vi "耐久性测试.vi"(6 "Bool引用句柄":refnum<vi>, 9 "输出簇 2":T4, 10 "输出簇":T4, 11 "事件注册引用句柄 2":refnum<event-registration>) -> ()   [LabVIEW 2020]
uses:
  <vilib>/Utility/miscctls.llb/LVRectTypeDef.ctl
  Windows/System32/user32.dll
panel:
  in  "布尔 3":T1
  in  "布尔 2":T2
  in  "布尔":T3
  out "数值 2":dbl format="%#_2f V"
  out "数值":dbl format="%#_2f A"
  out "电流":dbl[](graph)
  out "电压":dbl[](graph)
  # "耐久性测试"
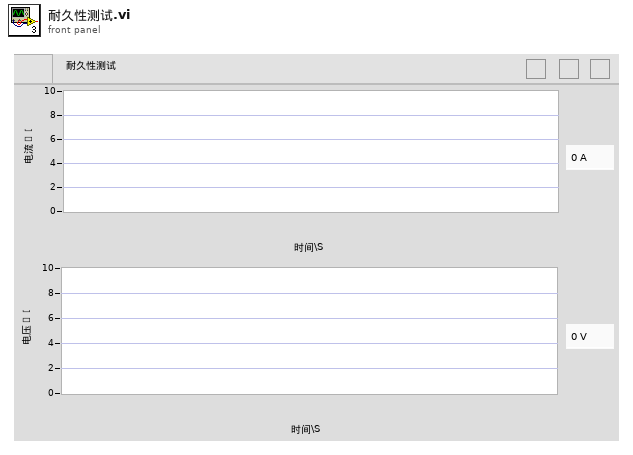
[diagram p1: front panel]
types:
  T1 = typedef "控件关闭.ctl" = bool
  T2 = typedef "控件最小化.ctl" = bool
  T3 = typedef "控件最大化.ctl" = bool
  T4 = cluster{"电流1":refnum<vi>, "电流2":refnum<vi>, "电流3":refnum<vi>, "电流4":refnum<vi>}
  T5 = typedef "LVRectTypeDef.ctl" = cluster{"Left":i16, "Top":i16, "Right":i16, "Bottom":i16}
  T6 = typedef "LVPoint32TypeDef.ctl" = cluster{"Horizontal":i32, "Vertical":i32}
  T7 = enum32{"Invalid", "Standard", "Closed", "Hidden", "Minimized", "Maximized"}
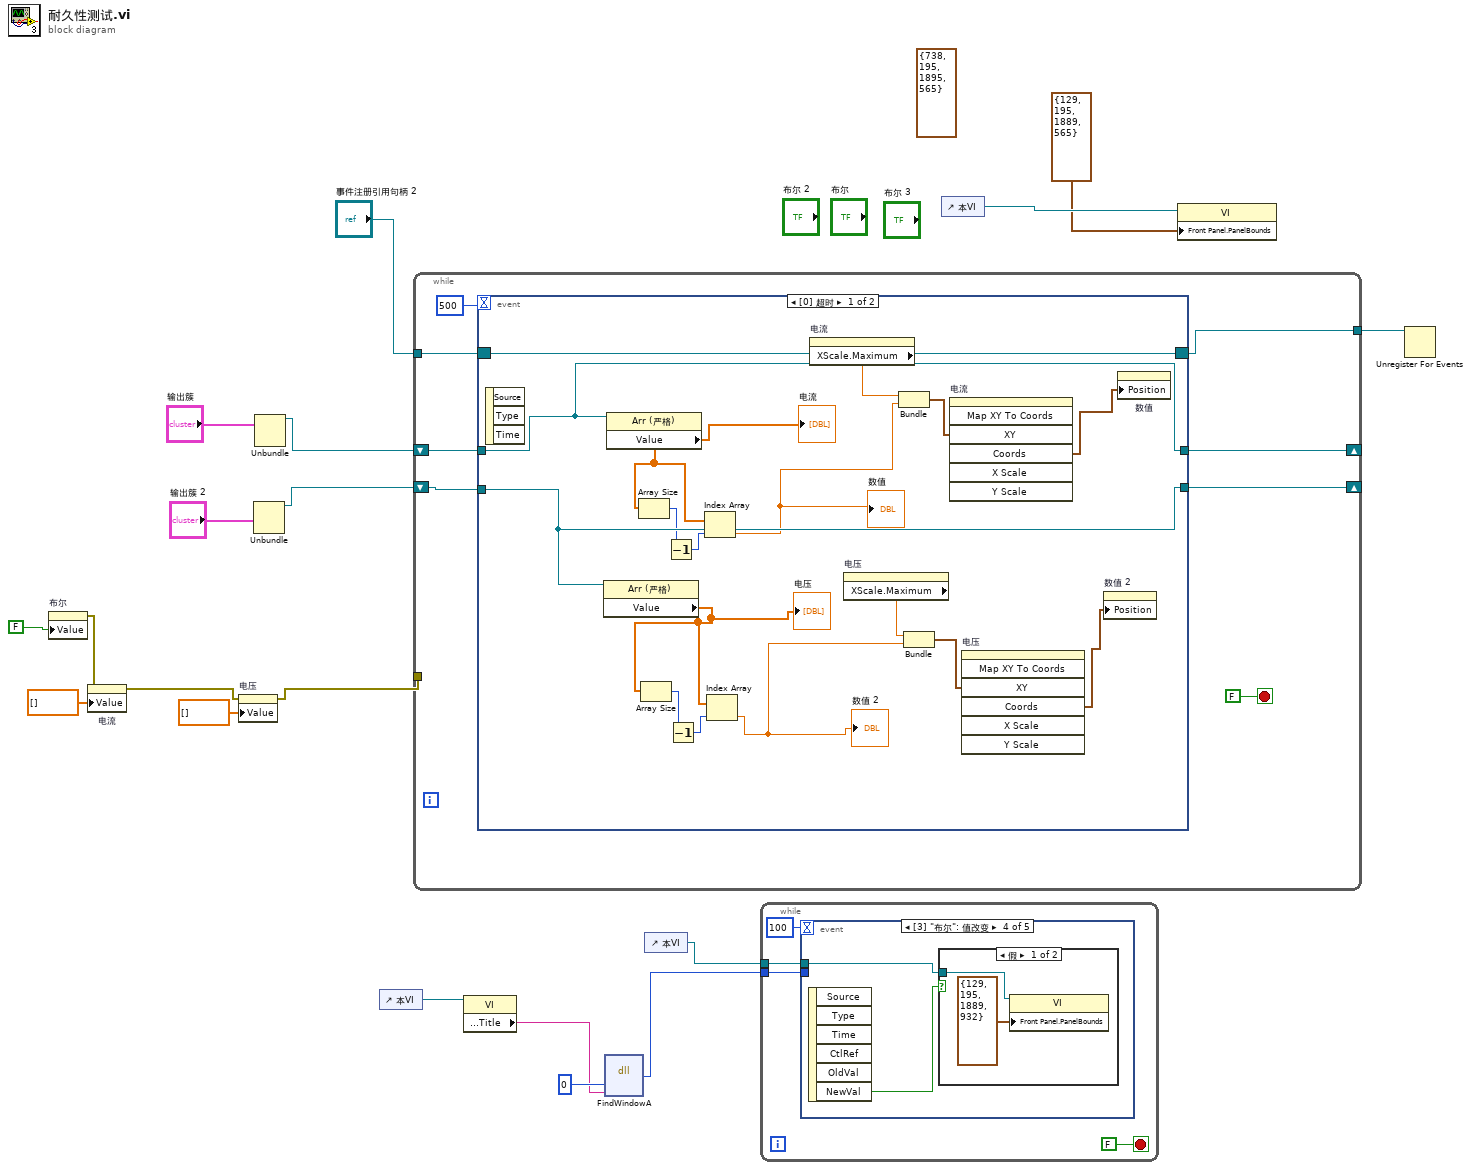
[diagram p0: block diagram]
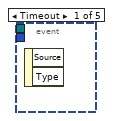
[diagram p2: hidden frame]
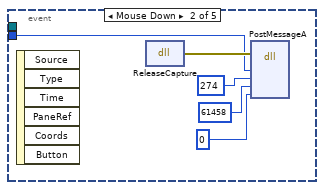
[diagram p3: hidden frame]
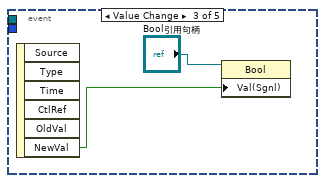
[diagram p4: hidden frame]
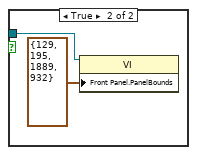
[diagram p5: hidden frame]
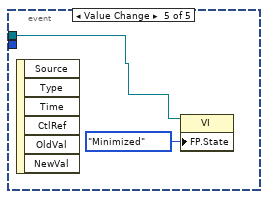
[diagram p6: hidden frame]
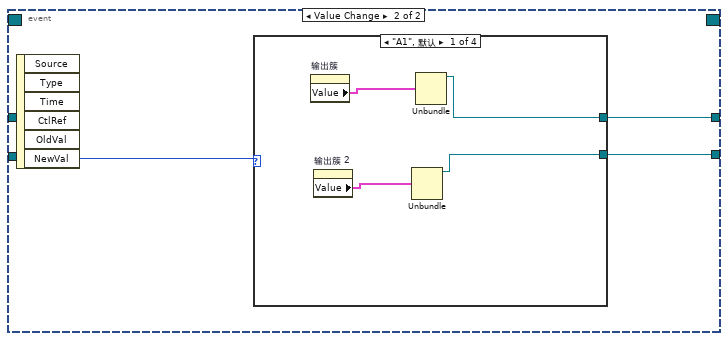
[diagram p7: hidden frame]
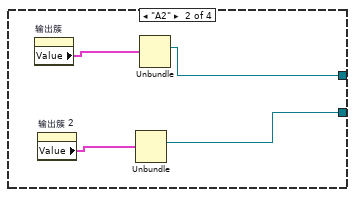
[diagram p8: hidden frame]
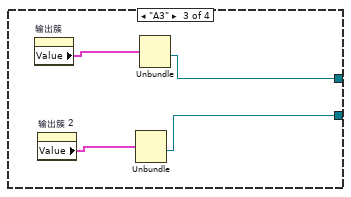
[diagram p9: hidden frame]
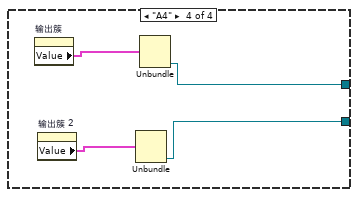
[diagram p10: hidden frame]
diagram:
  (unwired) T5 {"Left"=738, "Top"=195, "Right"=1895, "Bottom"=565} ("前面板窗口:前面板边界")
  n1 = property on="布尔" class="Bool (严格)"("Value"=T3 FALSE ("布尔")) -> (error out=w1:errorcluster)  [unwired: 2 in, 1 out]
  n2 = property on="电流" class="WFGraph (严格)"(error in=w1, "Value"=dbl[] [] ("电流")) -> (error out=w9:errorcluster)  [unwired: 1 in, 1 out]
  n3 = property on="电压" class="WFGraph (严格)"(error in=w9, "Value"=dbl[] [] ("电压")) -> (error out=w8:errorcluster)  [unwired: 1 in, 1 out]
  n4 = Unbundle("输出簇 2") -> ("电流1"=w3:refnum<vi>)  [unwired: 3 out]
  n5 = Unbundle("输出簇") -> ("电流1"=w4:refnum<vi>)  [unwired: 3 out]
  n6 = control-ref of="本VI"() -> (w17:refnum<vi>)
  n7 = while {
    tunnel: w8 -> [_]
    tunnel: "事件注册引用句柄 2" -> [w26]
    tunnel: [w25] -> w7
    shift-right: [w24] -> _
    shift-left: w4 -> [w22]
    shift-right: [w23] -> _
    shift-left: w3 -> [w21]
    stop <- FALSE stop-if-true
    n8 = event shown="[0] 超时" {
      selector: w26 -> [w44 _]
      dyn-events: [w44 _] -> w25
      timeout: 500 -> [_ _]
      tunnel: [w43 w46] -> w24
      tunnel: [w42 w45] -> w23
      tunnel: w22 -> [w43 _]
      tunnel: w21 -> [w42 _]
      event Timeout {
        n9 = event-data() -> ()  [unwired: 1 in, 3 out]
        n10 = property class="Arr (严格)"(reference=w42) -> ("Value"=w32:dbl[])  [unwired: 1 in, 2 out]
        "电压" <- w32
        n11 = property class="Arr (严格)"(reference=w43) -> ("Value"=w33:dbl[])  [unwired: 1 in, 2 out]
        "电流" <- w33
        n12 = Array Size(array=w33) -> (size(s)=w36:i32)
        n13 = Array Size(array=w32) -> (size(s)=w38:i32)
        n14 = Decrement(x=w36) -> (x-1=w35:i32)
        n15 = Decrement(x=w38) -> (x-1=w39:i32)
        n16 = Index Array(array=w33, index=w35) -> (element=w31:dbl)
        "数值" <- w31
        n17 = Index Array(array=w32, index=w39) -> (element=w30:dbl)
        "数值 2" <- w30
        n18 = property on="电流" class="WFGraph (严格)"() -> ("XScale.Maximum"=w41:dbl)  [unwired: 2 in, 2 out]
        n19 = property on="电压" class="WFGraph (严格)"() -> ("XScale.Maximum"=w40:dbl)  [unwired: 2 in, 2 out]
        n20 = Bundle("XScale.Maximum"=w41, "数值"=w31) -> (w34:cluster{"XScale.Maximum":dbl, "数值":dbl})  [unwired: 1 in]
        n21 = Bundle("XScale.Maximum"=w40, "数值"=w30) -> (w37:cluster{"XScale.Maximum":dbl, "数值":dbl})  [unwired: 1 in]
        n22 = invoke on="电流" class="WFGraph (严格)" method="Map XY To Coords"("XY"=w34) -> ("Coords"=w29:T6)  [unwired: 6 in, 6 out]
        n23 = invoke on="电压" class="WFGraph (严格)" method="Map XY To Coords"("XY"=w37) -> ("Coords"=w28:T6)  [unwired: 6 in, 6 out]
        n24 = property on="数值 2" class="DigNum (严格)"("Position"=w28) -> ()  [unwired: 2 in, 2 out]
        n25 = property on="数值" class="DigNum (严格)"("Position"=w29) -> ()  [unwired: 2 in, 2 out]
      }
      event Value Change {
        n26 = event-data() -> ("NewVal"=w47:enum32{"未选择", "A1", "A2", "A3", "A4"})  [unwired: 1 in, 5 out]
        n27 = case shown="\"A1\", 默认" w47 {
          tunnel: [w49 w53 w57 w60] -> w46
          tunnel: [w48 w52 w56 w61] -> w45
          frame "A1", Default {
            n28 = property on="输出簇" class="Clust (严格)"() -> ("Value"=w51:T4)  [unwired: 2 in, 2 out]
            n29 = property on="输出簇 2" class="Clust (严格)"() -> ("Value"=w50:T4)  [unwired: 2 in, 2 out]
            n30 = Unbundle(w50) -> ("电流1"=w48:refnum<vi>)  [unwired: 3 out]
            n31 = Unbundle(w51) -> ("电流1"=w49:refnum<vi>)  [unwired: 3 out]
          }
          frame "A2" {
            n32 = property on="输出簇" class="Clust (严格)"() -> ("Value"=w55:T4)  [unwired: 2 in, 2 out]
            n33 = property on="输出簇 2" class="Clust (严格)"() -> ("Value"=w54:T4)  [unwired: 2 in, 2 out]
            n34 = Unbundle(w54) -> ("电流2"=w52:refnum<vi>)  [unwired: 3 out]
            n35 = Unbundle(w55) -> ("电流2"=w53:refnum<vi>)  [unwired: 3 out]
          }
          frame "A3" {
            n36 = property on="输出簇" class="Clust (严格)"() -> ("Value"=w59:T4)  [unwired: 2 in, 2 out]
            n37 = property on="输出簇 2" class="Clust (严格)"() -> ("Value"=w58:T4)  [unwired: 2 in, 2 out]
            n38 = Unbundle(w58) -> ("电流3"=w56:refnum<vi>)  [unwired: 3 out]
            n39 = Unbundle(w59) -> ("电流3"=w57:refnum<vi>)  [unwired: 3 out]
          }
          frame "A4" {
            n40 = property on="输出簇" class="Clust (严格)"() -> ("Value"=w63:T4)  [unwired: 2 in, 2 out]
            n41 = property on="输出簇 2" class="Clust (严格)"() -> ("Value"=w62:T4)  [unwired: 2 in, 2 out]
            n42 = Unbundle(w62) -> ("电流4"=w61:refnum<vi>)  [unwired: 3 out]
            n43 = Unbundle(w63) -> ("电流4"=w60:refnum<vi>)  [unwired: 3 out]
          }
        }
      }
    }
  }
  n44 = property class="VI"(reference=w17) -> ("Front Panel.Title"=w16:string)  [unwired: 1 in, 2 out]
  n45 = dll-call lib="/Windows/System32/user32.dll" fn="FindWindowA"("lp"=u32 0, "name"=w16) -> ("返回类型"=w15:u32)  [unwired: 5 in, 2 out]
  n46 = control-ref of="本VI"() -> (w12:refnum<vi>)
  n47 = while {
    tunnel: w15 -> [w67]
    tunnel: w12 -> [w66]
    stop <- FALSE stop-if-true
    n48 = event shown="[3] \"布尔\": 值改变" {
      selector: _ -> [_ _ _ _ _]
      dyn-events: _ -> [_ _ _ _ _]
      timeout: 100 -> [_ _ _ _ _]
      tunnel: w67 -> [_ w68 _ _ _]
      tunnel: w66 -> [_ _ _ w75 w82]
      event Timeout {
        n49 = event-data() -> ()  [unwired: 1 in, 2 out]
      }
      event Mouse Down {
        n50 = event-data() -> ()  [unwired: 1 in, 6 out]
        n51 = dll-call lib="/Windows/System32/user32.dll" fn="ReleaseCapture"() -> (error out=w72:errorcluster)  [unwired: 4 in, 1 out]
        n52 = dll-call lib="/Windows/System32/user32.dll" fn="PostMessageA"(error in=w72, "lp"=w68, "name"=274, "vak"=61458, "val"=0) -> ()  [unwired: 7 in, 2 out]
      }
      event Value Change {
        n53 = event-data() -> ("NewVal"=w73:T1)  [unwired: 1 in, 5 out]
        n54 = property class="Bool"(reference="Bool引用句柄", "Val(Sgnl)"=w73) -> ()  [unwired: 1 in, 2 out]
      }
      event Value Change {
        n55 = event-data() -> ("NewVal"=w76:T3)  [unwired: 1 in, 5 out]
        n56 = case shown="假" w76 {
          tunnel: w75 -> [w78 w80]
          frame False {
            n57 = property class="VI"(reference=w78, "Front Panel.PanelBounds"=T5 {"Left"=129, "Top"=195, "Right"=1889, "Bottom"=932} ("前面板窗口:前面板边界")) -> ()  [unwired: 1 in, 2 out]
          }
          frame True {
            n58 = property class="VI"(reference=w80, "Front Panel.PanelBounds"=T5 {"Left"=129, "Top"=195, "Right"=1889, "Bottom"=932} ("前面板窗口:前面板边界")) -> ()  [unwired: 1 in, 2 out]
          }
        }
      }
      event Value Change {
        n59 = event-data() -> ()  [unwired: 1 in, 6 out]
        n60 = property class="VI"(reference=w82, "FP.State"=T7."Minimized" ("前面板窗口:状态")) -> ()  [unwired: 1 in, 2 out]
      }
    }
  }
  n61 = control-ref of="本VI"() -> (w19:refnum<vi>)
  n62 = property class="VI"(reference=w19, "Front Panel.PanelBounds"=T5 {"Left"=129, "Top"=195, "Right"=1889, "Bottom"=565} ("前面板窗口:前面板边界")) -> ()  [unwired: 1 in, 2 out]
  n63 = Unregister For Events(event registration refnum=w7) -> ()  [unwired: 1 in, 1 out]
